vi "Close.vi"(8 "error in (no error)":errorcluster, 11 "VISA resource name":refnum<visa-resource-name>) -> (0 "error out":errorcluster)   [LabVIEW 2011, in "Hokuyo URG Series.lvlib"]
doc: "Closes the session to the instrument. This VI ignores errors and attempts to always turn off the laser before terminating the software connection to the instrument."
uses:
  Hokuyo URG Series.lvlib
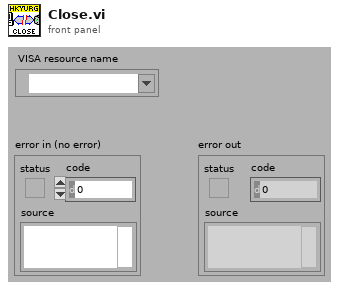
[diagram p1: front panel]
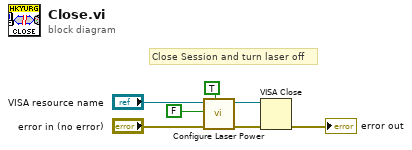
[diagram p0: block diagram]
diagram:
  # "Close Session and turn laser off"
  n1 = call "Configure Laser Power.vi"("Ignore Errors"=TRUE, "error in (no error)"="error in (no error)", "Laser Power"=FALSE ("Laser"), "VISA resource name"="VISA resource name") -> ("error out"=w4:errorcluster, "VISA resource name out"=w3:refnum<visa-resource-name>)  [unwired: 6 in]
  n2 = VISA Close(VISA resource name=w3, error in (no error)=w4) -> (error out=→"error out":errorcluster)
